vi "TestExec.Result, Meas Limit Check.vi"(10 "Test Limit":T3, 11 "Meas In":T2 {"Status" items=["LOG", "PASS", "FAIL", "ERROR"]}) -> (3 "Meas Out":T2 {"Status" items=["LOG", "PASS", "FAIL", "ERROR"]})   [LabVIEW 2019]
uses:
  Results/Limits/Result.Test Limit Item.ctl
  Results/Result.Limit Type.ctl
  Results/Result.Measurement Item.ctl
  Results/Result.Measurement and Attribute Item Status.ctl
panel:
  out "Status":T1 items=["LOG", "PASS", "FAIL", "ERROR"]
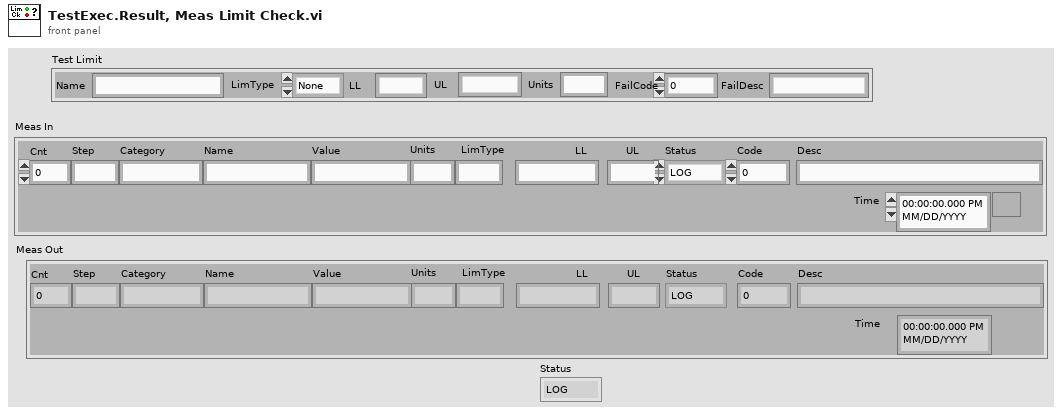
[diagram p1: front panel]
types:
  T1 = typedef "Result.Measurement and Attribute Item Status.ctl" = i32
  T2 = typedef "Result.Measurement Item.ctl" = cluster{"Cnt":i32, "Step":string, "Category":string, "Name":string, "Value":string, "Units":string, "LimType":string, "LL":string, "UL":string, "Status":T1, "Code":i32, "Desc":string, "Time":timestamp}
  T3 = typedef "Result.Test Limit Item.ctl" = cluster{"Name":string, "LimType":T4, "LL":string, "UL":string, "Units":string, "FailCode":i32, "FailDesc":string}
  T4 = typedef "Result.Limit Type.ctl" = enum16{"None", "EQ", "NE", "GT", "LT", "GE", "LE", "GTLT", "GELE", "GELT", "GTLE", "LTGT", "LEGE", "LEGT", "LTGE", "Contains", "NotContains"}
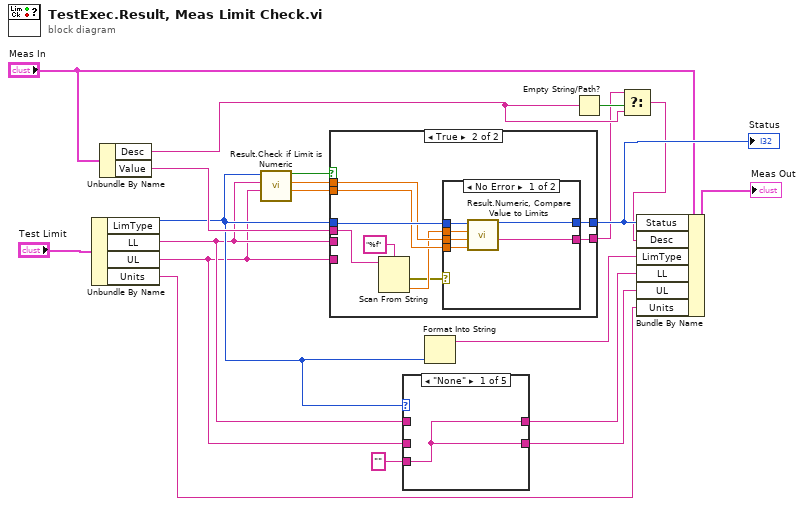
[diagram p0: block diagram]
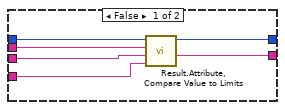
[diagram p6: hidden frame]
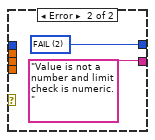
[diagram p7: hidden frame]
diagram:
  n1 = Unbundle By Name("Test Limit") -> ("LimType"=w9:T4, "LL"=w8:string, "UL"=w7:string, "Units"=w14:string)
  n2 = Unbundle By Name("Meas In") -> ("Desc"=w12:string, "Value"=w20:string)
  n3 = call "Result.Check if Limit is Numeric.vi"("UL"=w7, "LL"=w8, "LimType"=w9) -> ("UL Num"=w4:dbl, "LL Num"=w5:dbl, "Is Numeric"=w6:bool)  [unwired: 6 in]
  n4 = case shown="True" w6 {
    tunnel: [w26 w35] -> w19
    tunnel: w9 -> [w25 w34]
    tunnel: w8 -> [w24 _]
    tunnel: w7 -> [w23 _]
    tunnel: [w22 w27] -> w11
    tunnel: w20 -> [w21 w32]
    tunnel: w5 -> [_ w31]
    tunnel: w4 -> [_ w30]
    frame False {
      n5 = call "Result.Attribute, Compare Value to Limits.vi"("UL"=w23, "LL"=w24, "Value"=w21, "LimType"=w25) -> ("Desc"=w22:string, "Status"=w26:T1)  [unwired: 6 in]
    }
    frame True {
      n6 = Scan From String(format string="%f", input string=w32) -> (error out=w28:errorcluster, output 1=w29:dbl)  [unwired: 3 in, 2 out]
      n7 = case shown="No Error" w28 {
        tunnel: [w41 w43] -> w35
        tunnel: w34 -> [w40 _]
        tunnel: w31 -> [w39 _]
        tunnel: w30 -> [w38 _]
        tunnel: w29 -> [w37 _]
        tunnel: [w36 "Value is not a number and limit check is numeric." ("Desc")] -> w27
        frame No Error {
          n8 = call "Result.Numeric, Compare Value to Limits.vi"("UL"=w38, "LL"=w39, "Value"=w37, "LimType"=w40) -> ("Desc"=w36:string, "Status"=w41:T1)  [unwired: 6 in]
        }
        frame Error {
          w43 = T1 2 items=["LOG", "PASS", "FAIL", "ERROR"] ("Status")
        }
      }
    }
  }
  "Status" <- w19
  n9 = case shown="\"None\"" w9 {
    tunnel: w8 -> [_ w46 w48 _ w51]
    tunnel: w7 -> [_ _ _ w49 w52]
    tunnel: "" -> [w44 w45 w47 w50 _]
    tunnel: [w44 w46 w48 w50 w51] -> w16
    tunnel: [w44 w45 w47 w49 w52] -> w15
    frame "None" {
    }
    frame "EQ".."GT", "GE" {
    }
    frame "Contains", "NotContains" {
    }
    frame "LT", "LE" {
    }
    frame Default {
    }
  }
  n10 = Format Into String(w9) -> (resulting string=w18:string)  [unwired: 3 in, 1 out]
  n11 = Empty String/Path?(string/path=w12) -> (empty?=w13:bool)
  n12 = Select(t=w11, s=w13, f=w12) -> (s? t:f=w10:string)
  n13 = Bundle By Name(cluster="Meas In", "Status"=w19, "Desc"=w10, "LimType"=w18, "LL"=w16, "UL"=w15, "Units"=w14) -> (→"Meas Out":T2)
